vi "findPHSerror.vi"() -> ()   [LabVIEW 2016]
uses:
  <vilib>/Utility/file.llb/Write Delimited Spreadsheet (DBL).vi
panel:
  in  "osc in":refnum<visa-resource-name>
  out "Real":dbl
  in  "freq (MHz)":dbl=1.367
  in  "HIFU port":u32=12321
  in  "HIFU ip":string="192.168.1.24"
  out "Waveform Graph":dbl[](graph)
  out "channel":dbl
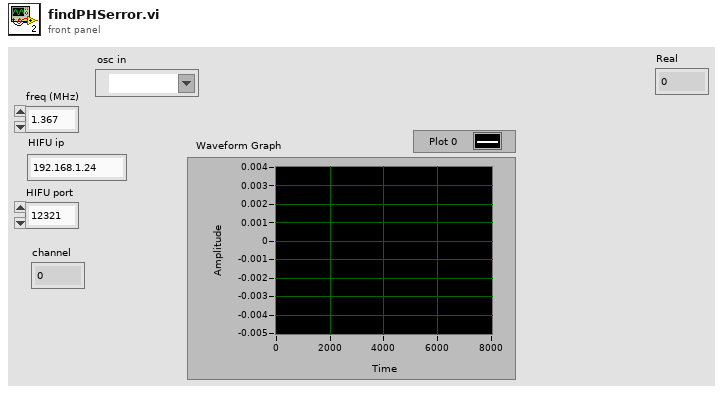
[diagram p1: front panel]
types:
  T1 = typedef "NI_Matrix.lvlib/RealMatrix.ctl" = dbl[][]
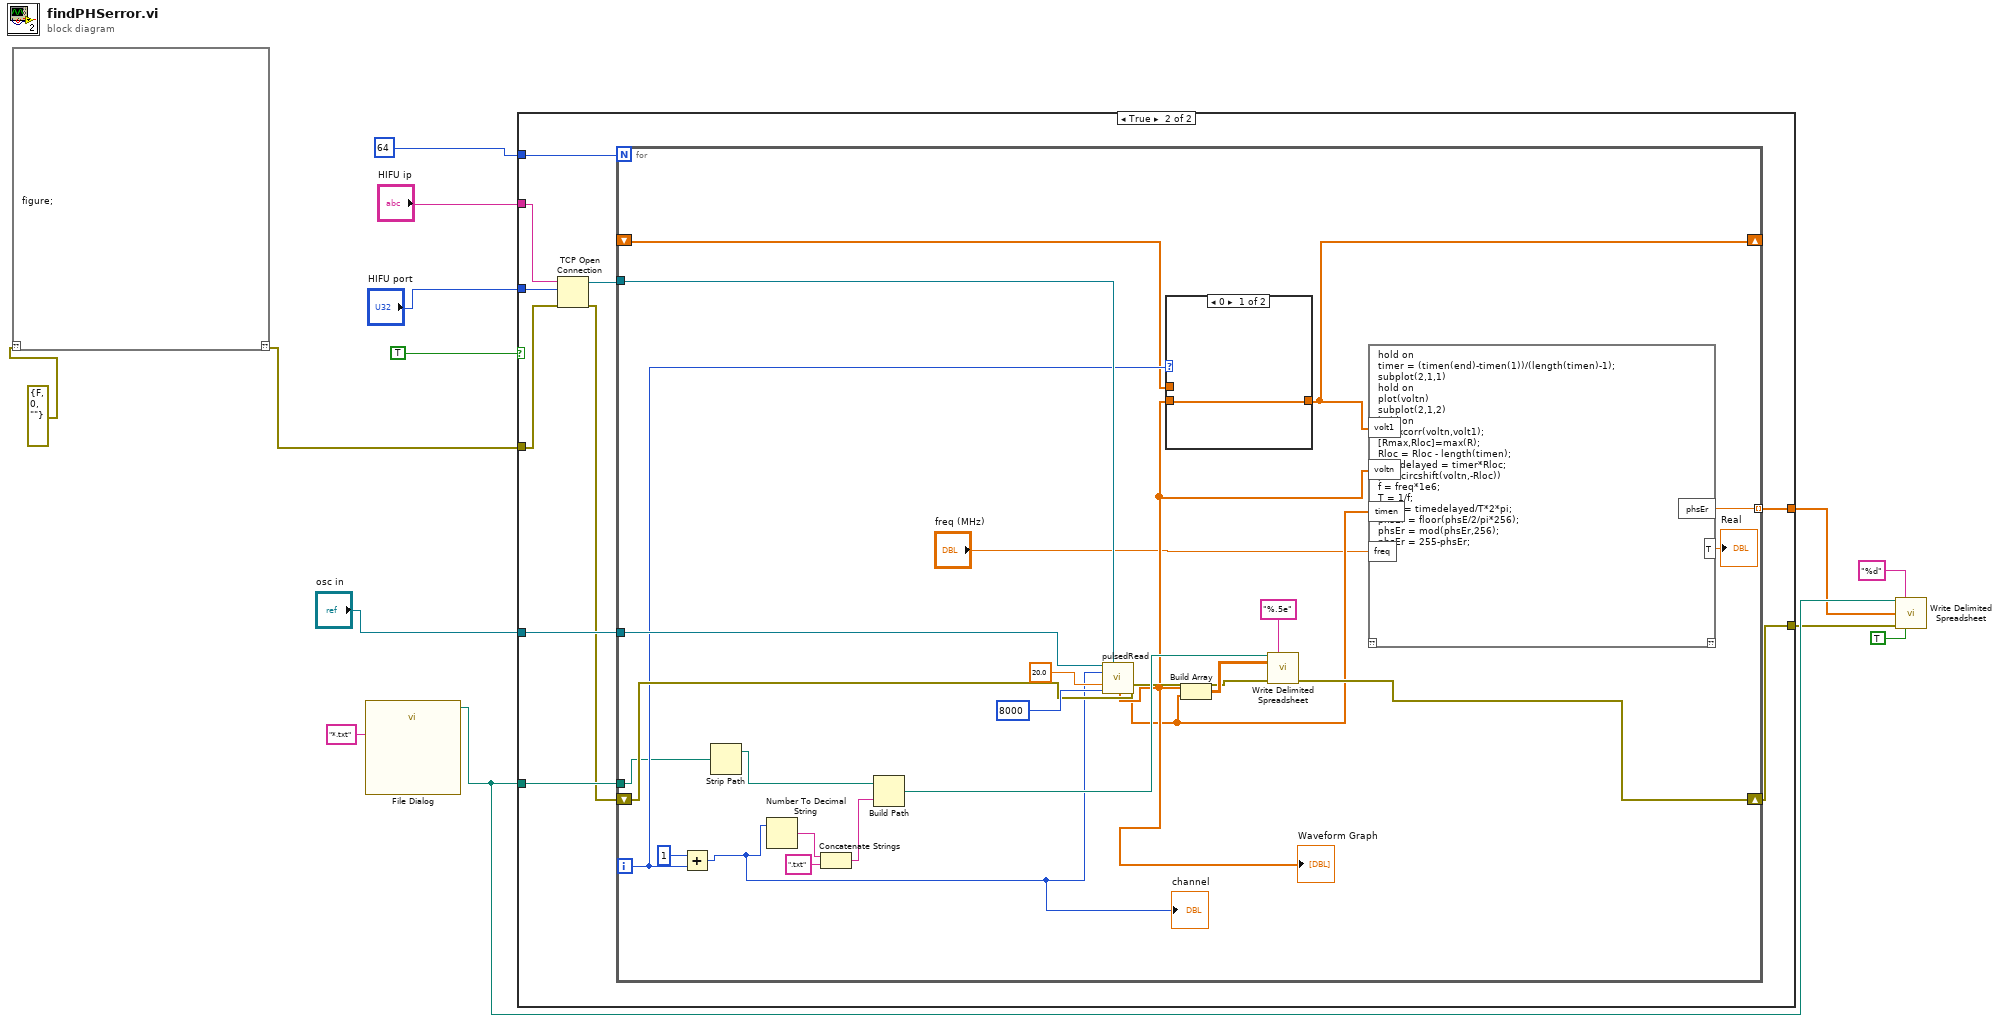
[diagram p0: block diagram]
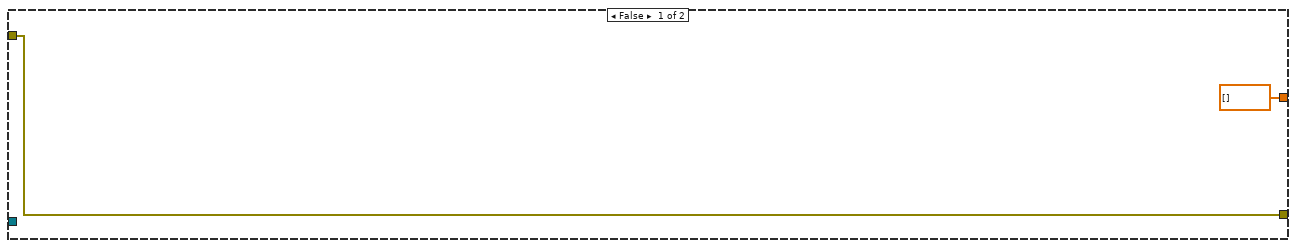
[diagram p2: hidden frame]
diagram:
  n1 = script code="figure;"("??"=errorcluster {"status"=FALSE, "code"=0, "source"=""} ("error out")) -> ("??"=w1:errorcluster)
  n2 = call "File Dialog"("pattern (all files)"="*.txt") -> ("selected path"=w7:path)  [unwired: 11 in, 3 out]
  n3 = case shown="True" TRUE {
    tunnel: 64 -> [_ w25]
    tunnel: w1 -> [w14 w20]
    tunnel: "osc in" -> [_ w24]
    tunnel: w7 -> [_ w23]
    tunnel: "HIFU ip" -> [_ w22]
    tunnel: "HIFU port" -> [_ w21]
    tunnel: [dbl[] [] w17] -> w6
    tunnel: [w14 w16] -> w5
    frame False {
    }
    frame True {
      n4 = TCP Open Connection(address=w22, remote port or service name=w21, error in (no error)=w20) -> (connection ID=w18:refnum<k5>, error out=w19:errorcluster)  [unwired: 2 in]
      n5 = for {
        N: w25 -> [_]
        tunnel: w24 -> [w40]
        tunnel: w23 -> [w28]
        shift-right: [w39] -> w16
        shift-left: w19 -> [w41]
        tunnel: w18 -> [w37]
        shift-right: [w33] -> _
        shift-left: _ -> [w34]
        tunnel: [w29] -> w17 mode=indexing
        i -> [w35]
        n6 = Add(x=1, y=w35) -> (x+y=w36:i32)
        "channel" <- w36
        n7 = Strip Path(path=w28) -> (stripped path=w27:path)  [unwired: 1 out]
        n8 = Number To Decimal String(number=w36) -> (decimal integer string=w46:string)  [unwired: 1 in]
        n9 = Concatenate Strings(w46, ".txt" ("string")) -> (w45:string)
        n10 = Build Path(base path=w27, name or relative path=w45) -> (appended path=w44:path)
        n11 = call "pulsedRead.vi"("osc in"=w40, "connection ID"=w37, "channel"=w36, "error in (no error)"=w41, "cycles"=20.0, "points"=u64 8000) -> ("error out"=w42:errorcluster, "voltage"=w32:dbl[], "time"=w31:dbl[])  [unwired: 4 in, 3 out]
        "Waveform Graph" <- w32
        n12 = case shown="0" w35 {
          tunnel: w32 -> [w51 _]
          tunnel: [w51 w52] -> w33
          tunnel: w34 -> [_ w52]
          frame 0 {
          }
          frame 1, Default {
          }
        }
        n13 = Build Array(w32, w31) -> (w43:T1)
        n14 = call-poly <vilib>:"Write Delimited Spreadsheet.vi"("file path (dialog if empty)"=w44, "format (%.3f)"="%.5e", "2D data"=w43, "error in (no error)"=w42) -> ("error out"=w39:errorcluster)  [unwired: 10 in, 1 out]
        n15 = script code="hold on\ntimer = (timen(end)-timen(1))/(length(timen)-1);\nsubplot(2,1,1)\nhold on\nplot(voltn)\nsubplot(2,1,2)\nhold on\nR = xcorr(voltn,volt1);\n[Rmax,Rloc]=max(R);\nRloc = Rloc - length(timen);\ntimedelayed = timer*Rloc;\nplot(circshift(voltn,-Rloc))\nf = freq*1e6;\nT = 1/f;\nphsE = timedelayed/T*2*pi;\nphsEr = floor(phsE/2/pi*256);\nphsEr = mod(phsEr,256);\nphsEr = 255-phsEr;"("volt1"=w33, "voltn"=w32, "timen"=w31, "freq"="freq (MHz)") -> ("phsEr"=w29:dbl, "T"=→"Real":dbl)  [unwired: 1 in, 1 out]
      }
    }
  }
  n16 = call-poly <vilib>:"Write Delimited Spreadsheet.vi"("file path (dialog if empty)"=w7, "format (%.3f)"="%d", "1D data"=w6, "error in (no error)"=w5, "transpose? (no:F)"=TRUE) -> ()  [unwired: 9 in, 2 out]
